vi "prepare dark model.vi"(8 "error in (no error)":errorcluster, 11 "Settings in":T1={"Hardware Configuration"={"AVS Settings"={"Communication Settings"={"Serial1"="", "Handle1"=0, "a_pDeviceId1"=[], "a_pNumPixels"=0, "Port"=0, "a_hWnd"=0}, "a_pMeasConfig1"={"StartPixel"=0, "StopPixel"=0, "IntTime"=0.0, "IntDelay"=0, "NrOfAVG"=0, "DarkEnable"=0, "ForgetPercentage"=0, "SmoothPix"=0, "SmoothModel"=0, "SatDetection"=0, "TriggerMode"=0, "TriggerSource"=0, "TriggerSourceType"=0, "FlashesPerScan"=0, "LaserDelay"=0, "LaserWidth"=0, "LaserWavelenght"=0.0, "RamSpectra"=0}, "Dark Correct"=FALSE, "Auto Determine Int Time"=FALSE}, "Sphere Indicator"=enum."Naked Sphere", "Measurement Type"=enum."Normal", "Correction Files"={"Calibration File"=path "", "Cal lamp in, cal lamp on"=path "", "Cal lamp in, aux lamp on"=path "", "DUT in, aux lamp on"=path "", "Dark Model"=path "C:/Users/dhstuart/Dropbox/CLTC/avantesSpectrometer/Settings/Naked Sphere/Cal Files/Dark Array2015_4_15_.csv", "Dark Array"=path ""}}, "Logging Configuration"={"Log File Base Path"=path "", "Cal File Folder"=path "", "TDMS File Reference"=refnum}, "Base Path"=path "C:/Users/dhstuart/Dropbox/CLTC/avantesSpectrometer"}) -> (0 "error out":errorcluster, 3 "Settings in out":T1={"Hardware Configuration"={"AVS Settings"={"Communication Settings"={"Serial1"="", "Handle1"=0, "a_pDeviceId1"=[], "a_pNumPixels"=0, "Port"=0, "a_hWnd"=0}, "a_pMeasConfig1"={"StartPixel"=0, "StopPixel"=0, "IntTime"=0.0, "IntDelay"=0, "NrOfAVG"=0, "DarkEnable"=0, "ForgetPercentage"=0, "SmoothPix"=0, "SmoothModel"=0, "SatDetection"=0, "TriggerMode"=0, "TriggerSource"=0, "TriggerSourceType"=0, "FlashesPerScan"=0, "LaserDelay"=0, "LaserWidth"=0, "LaserWavelenght"=0.0, "RamSpectra"=0}, "Dark Correct"=FALSE, "Auto Determine Int Time"=FALSE}, "Sphere Indicator"=enum."Naked Sphere", "Measurement Type"=enum."Normal", "Correction Files"={"Calibration File"=path "", "Cal lamp in, cal lamp on"=path "", "Cal lamp in, aux lamp on"=path "", "DUT in, aux lamp on"=path "", "Dark Model"=path "C:/Users/dhstuart/Dropbox/CLTC/avantesSpectrometer/Settings/Naked Sphere/Cal Files/Dark Array2015_4_15_.csv", "Dark Array"=path ""}}, "Logging Configuration"={"Log File Base Path"=path "", "Cal File Folder"=path "", "TDMS File Reference"=refnum}, "Base Path"=path "C:/Users/dhstuart/Dropbox/CLTC/avantesSpectrometer"})   [LabVIEW 2014, in "AvaSpec.lvlib" / "Dark.lvlib"]
uses:
  Dark.lvlib
  Settings/Settings.ctl
  Acquisition/Hardware Configuration.ctl
  Libraries/AS-5216-DLL/AVS settings.ctl
  Acquisition/Sphere Indicator.ctl
  Settings/Measurement Type.ctl
  Logging/Logging Configuration.ctl
  <vilib>/Analysis/baseanly.llb/Mean (DBL).vi
  <vilib>/Utility/file.llb/Write To Spreadsheet File (DBL).vi
  <vilib>/Analysis/NI_AALBase.lvlib
  Settings/AvaSpec Settings.lvlib
  AvaSpec.lvlib
  Acquisition/AvaSpec Acquisition.lvlib
  Logging/AvaSpec Logging.lvlib
panel:
  out "Intercept Fit Verification":cluster{dbl[], "Best Power Fit":dbl[]}[](graph)
  out "Slope Fit Verification":cluster{dbl[], "Best Power Fit":dbl[]}[](graph)
  out "Offset Power model":dbl[](array[numeric])
  out "Slope Power model":dbl[](array[numeric])
  out "Average Residuals":dbl[](array[numeric])
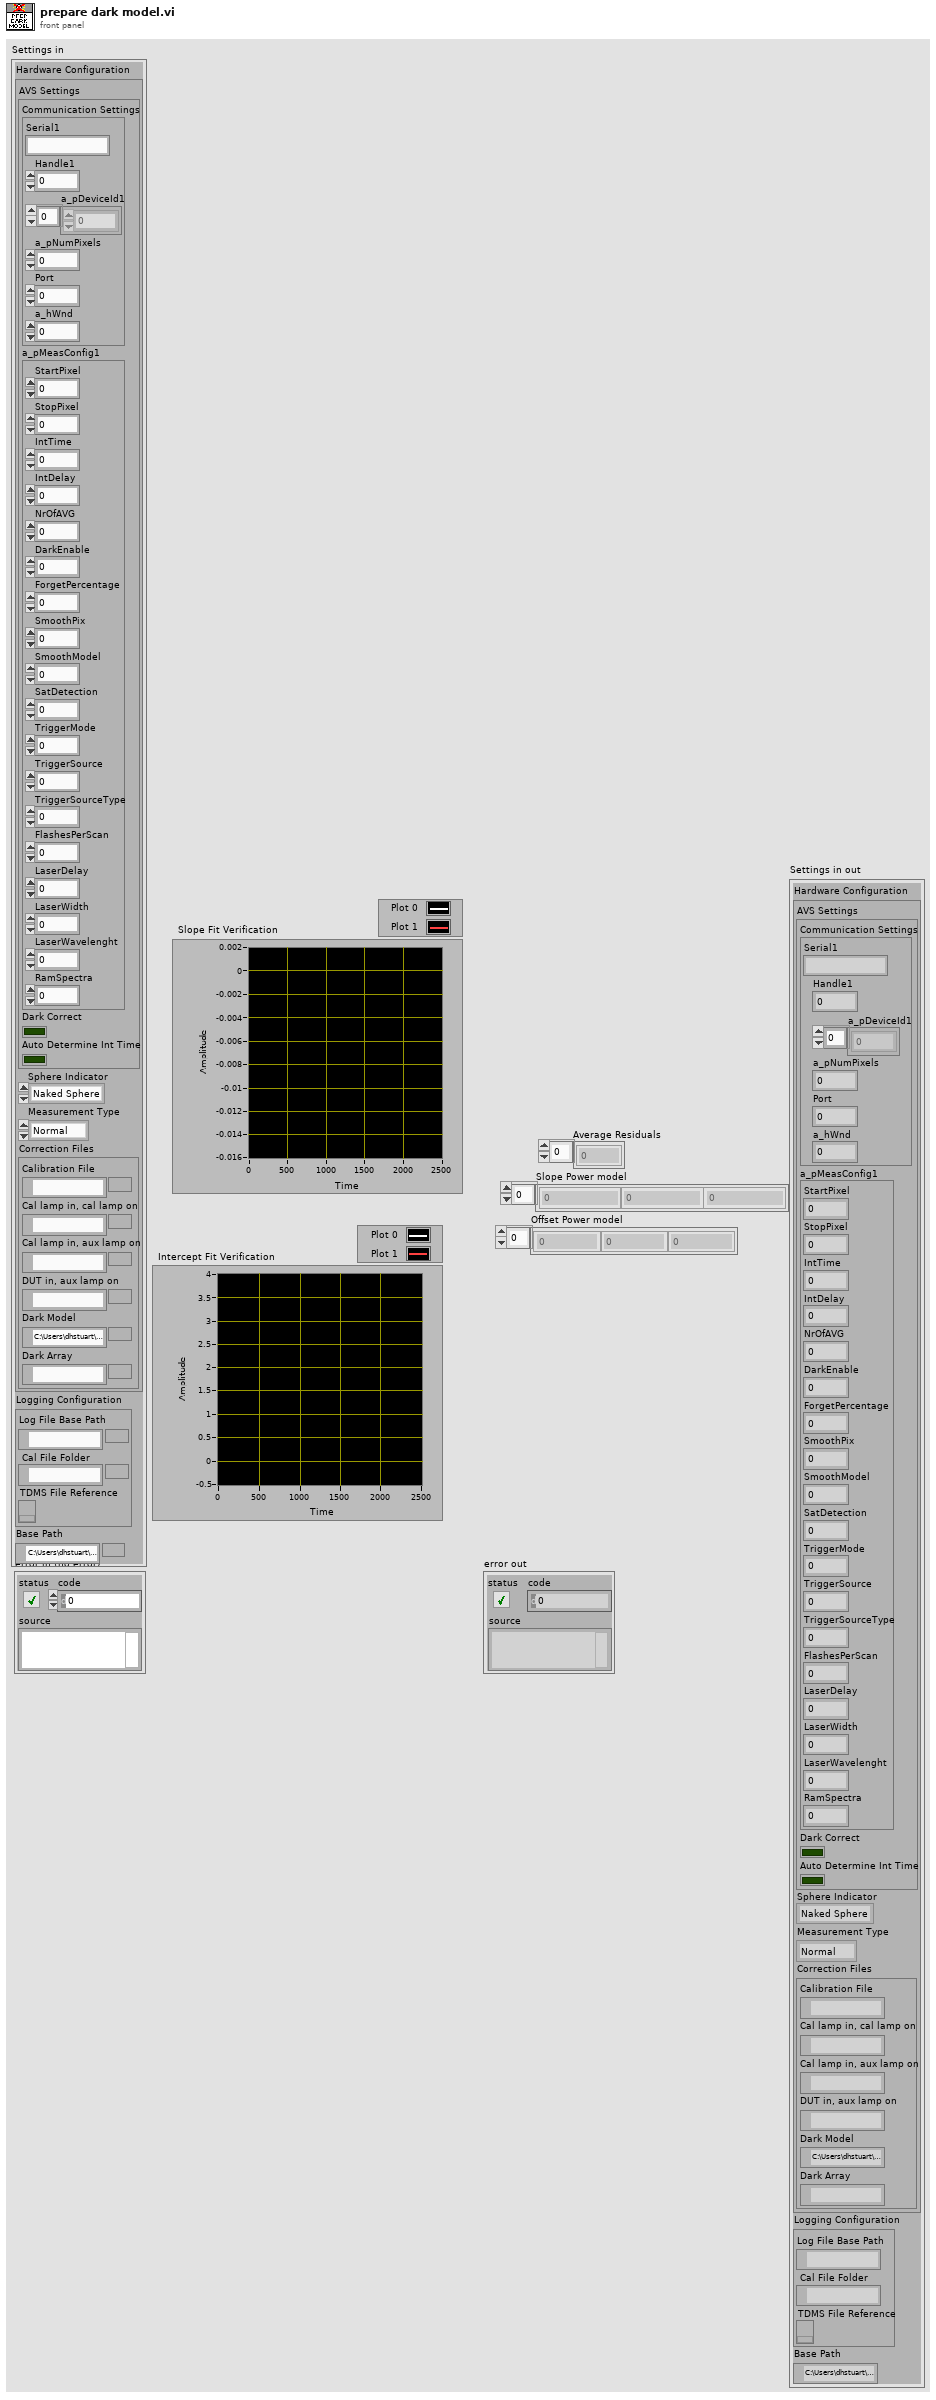
[diagram p1: front panel]
types:
  T1 = typedef "AvaSpec.lvlib/AvaSpec Settings.lvlib/Settings.ctl" = cluster{"Hardware Configuration":T2, "Logging Configuration":T6, "Base Path":path}
  T2 = typedef "AvaSpec.lvlib/AvaSpec Acquisition.lvlib/Hardware Configuration.ctl" = cluster{"AVS Settings":T3, "Sphere Indicator":T4, "Measurement Type":T5, "Correction Files":cluster{"Calibration File":path, "Cal lamp in, cal lamp on":path, "Cal lamp in, aux lamp on":path, "DUT in, aux lamp on":path, "Dark Model":path, "Dark Array":path}}
  T3 = typedef "AvaSpec.lvlib/AVS settings.ctl" = cluster{"Communication Settings":cluster{"Serial1":string, "Handle1":i32, "a_pDeviceId1":u8[], "a_pNumPixels":u16, "Port":i32, "a_hWnd":i32}, "a_pMeasConfig1":cluster{"StartPixel":u16, "StopPixel":u16, "IntTime":sgl, "IntDelay":u32, "NrOfAVG":u32, "DarkEnable":u8, "ForgetPercentage":u8, "SmoothPix":u16, "SmoothModel":u8, "SatDetection":u8, "TriggerMode":u8, "TriggerSource":u8, "TriggerSourceType":u8, "FlashesPerScan":u16, "LaserDelay":u32, "LaserWidth":u32, "LaserWavelenght":sgl, "RamSpectra":u16}, "Dark Correct":bool, "Auto Determine Int Time":bool}
  T4 = typedef "AvaSpec.lvlib/Sphere Indicator.ctl" = enum16{"Naked Sphere", "Insulated Sphere"}
  T5 = typedef "AvaSpec.lvlib/AvaSpec Acquisition.lvlib/Measurement Type.ctl" = enum16{"Normal", "Calibration", "Dark"}
  T6 = typedef "AvaSpec.lvlib/AvaSpec Logging.lvlib/Logging Configuration.ctl" = cluster{"Log File Base Path":path, "Cal File Folder":path, "TDMS File Reference":refnum<k34>}
  T7 = cluster{"amp min":dbl, "amp max":dbl, "power min":dbl, "power max":dbl, "offset min":dbl, "offset max":dbl}
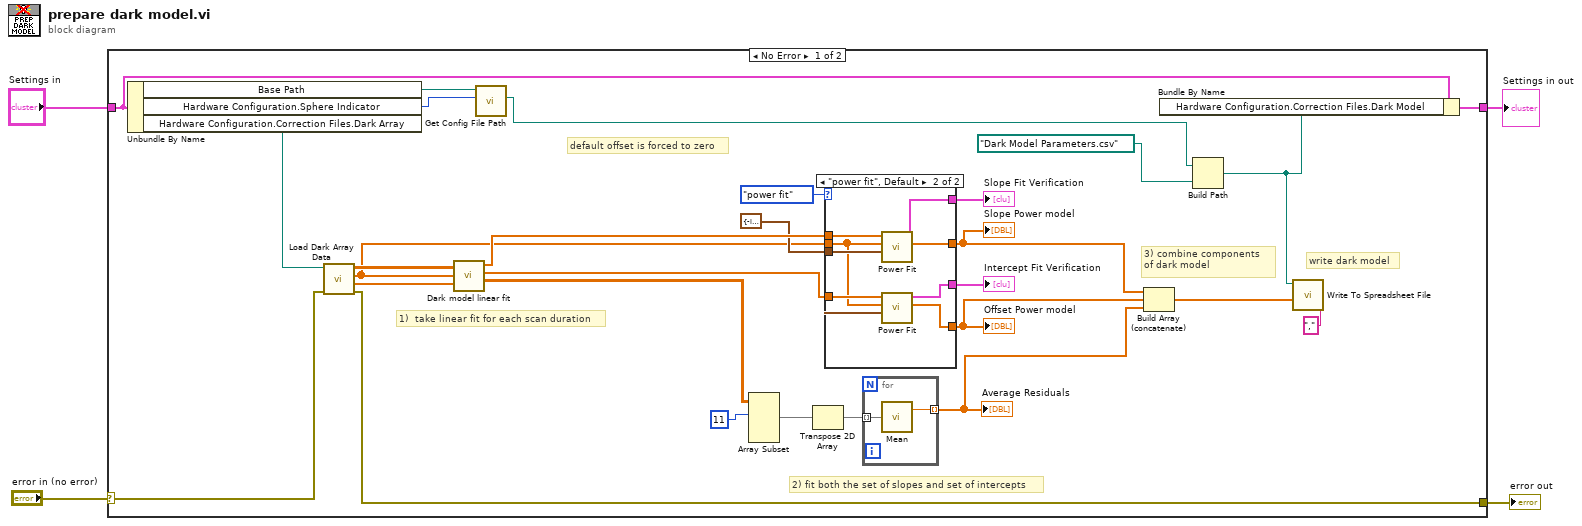
[diagram p0: block diagram]
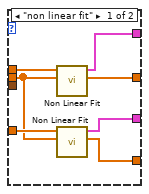
[diagram p2: hidden frame]
diagram:
  n1 = case shown="No Error" "error in (no error)" {
    selector: "error in (no error)" -> [w10 w51]
    tunnel: [w9 w51] -> w3
    tunnel: "Settings in" -> [w8 w50]
    tunnel: [w7 w50] -> w1
    frame No Error {
      # "3) combine components\nof dark model"
      # "write dark model"
      # "2) fit both the set of slopes and set of intercepts"
      # "1)  take linear fit for each scan duration"
      # "default offset is forced to zero"
      n2 = Unbundle By Name(w8) -> ("Base Path"=w15:path, "Hardware Configuration.Sphere Indicator"=w14:T4, "Hardware Configuration.Correction Files.Dark Array"=w11:path)
      n3 = call "Load Dark Array Data.vi"("error in (no error)"=w10, "Dark Array Path"=w11) -> ("error out"=w9:errorcluster, "Freq"=w27:dbl[], "intTime"=w16:dbl[], "Scans"=w32:dbl[][])  [unwired: 6 in]
      n4 = call "Dark model linear fit.vi"("Frequencies"=w27, "Integration Times"=w16, "Scans"=w32) -> ("Residuals"=w31:dbl[][], "Intercepts"=w20:dbl[], "Slopes"=w26:dbl[])  [unwired: 6 in]
      n5 = call "Get Config File Path.vi"("Sphere indicator"=w14, "Base Path"=w15) -> ("Cal File Folder"=w13:path)  [unwired: 7 in, 2 out]
      n6 = Array Subset(array=w31, index (row)=11 ("index")) -> (w23:dbl[][])  [unwired: 3 in]
      n7 = Transpose 2D Array(2D array=w23) -> (transposed array=w22:dbl[][])
      n8 = case shown="\"power fit\", Default" enum16{"non linear fit", "power fit"}."power fit" {
        tunnel: [w36 w47] -> w30
        tunnel: w26 -> [w35 w46]
        tunnel: [w37 w45] -> w25
        tunnel: w20 -> [w34 w44]
        tunnel: T7 {"amp min"=-inf, "amp max"=inf, "power min"=-inf, "power max"=inf, "offset min"=-10.0, "offset max"=10.0} ("parameter bounds") -> [_ w43]
        tunnel: [w39 w42] -> w18
        tunnel: [w38 w41] -> w17
        tunnel: w16 -> [w33 w40]
        frame "non linear fit" {
          n9 = call "Non Linear Fit.vi"("Integration Times"=w33, "Slopes"=w35) -> ("Non Linear Model"=w36:dbl[], "Fit Verification"=w37:cluster{dbl[], "Best Power Fit":dbl[]}[])  [unwired: 8 in]
          n10 = call "Non Linear Fit.vi"("Integration Times"=w33, "Slopes"=w34) -> ("Non Linear Model"=w38:dbl[], "Fit Verification"=w39:cluster{dbl[], "Best Power Fit":dbl[]}[])  [unwired: 8 in]
        }
        frame "power fit", Default {
          n11 = call "Power Fit.vi"("parameter bounds"=w43, "Integration Times"=w40, "Slopes"=w46) -> ("Power Model"=w47:dbl[], "Fit Verification"=w45:cluster{dbl[], "Best Power Fit":dbl[]}[])  [unwired: 7 in]
          n12 = call "Power Fit.vi"("parameter bounds"=w43, "Integration Times"=w40, "Slopes"=w44) -> ("Power Model"=w41:dbl[], "Fit Verification"=w42:cluster{dbl[], "Best Power Fit":dbl[]}[])  [unwired: 7 in]
        }
      }
      "Slope Power model" <- w30
      "Offset Power model" <- w17
      "Slope Fit Verification" <- w25
      "Intercept Fit Verification" <- w18
      n13 = for {
        tunnel: w22 -> [w49] mode=indexing
        tunnel: [w48] -> w21 mode=indexing
        n14 = call-poly <vilib>:"Mean.vi"("X"=w49) -> ("mean"=w48:dbl)  [unwired: 1 out]
      }
      "Average Residuals" <- w21
      n15 = Build Array (concatenate)(w30, w17, w21) -> (w29:dbl[])
      n16 = Build Path(base path=w13, name or relative path=path "Dark Model Parameters.csv" ("file path (dialog if empty)")) -> (appended path=w6:path)
      n17 = Bundle By Name(cluster=w8, "Hardware Configuration.Correction Files.Dark Model"=w6) -> (w7:T1)
      n18 = call-poly <vilib>:"Write To Spreadsheet File.vi"("delimiter (\\t)"="," ("delimiter (\\t)"), "1D data"=w29, "file path (dialog if empty)"=w6) -> ()  [unwired: 5 in, 1 out]
    }
    frame Error {
    }
  }
  "error out" <- w3
  "Settings in out" <- w1
